vi "Periodic Tasks.vi"() -> ()   [LabVIEW 2019]
doc: "This VI runs in parallel to other tasks. It can contain as many user-defined periodic loops as you need. These can carry out PID or other sorts of timed response."
uses:
  <vilib>/Rock Robotics/Network Tables/NT Write Raw.vi
  Robot Global Data.vi
  <vilib>/vision/Image Controls.llb/IMAQ Image.ctl
  <vilib>/Rock Robotics/WPI/RobotDrive/WPI_RobotDriveArcadeDrive_Standard(NoSaturation).vi
panel:
  in  "Y axis value":dbl
  in  "X axis value":dbl
  in  "Shooting Bottom Output":dbl
  in  "Shooting Top Output":dbl
  in  "Transport Output":dbl
  in  "Intake Output":dbl
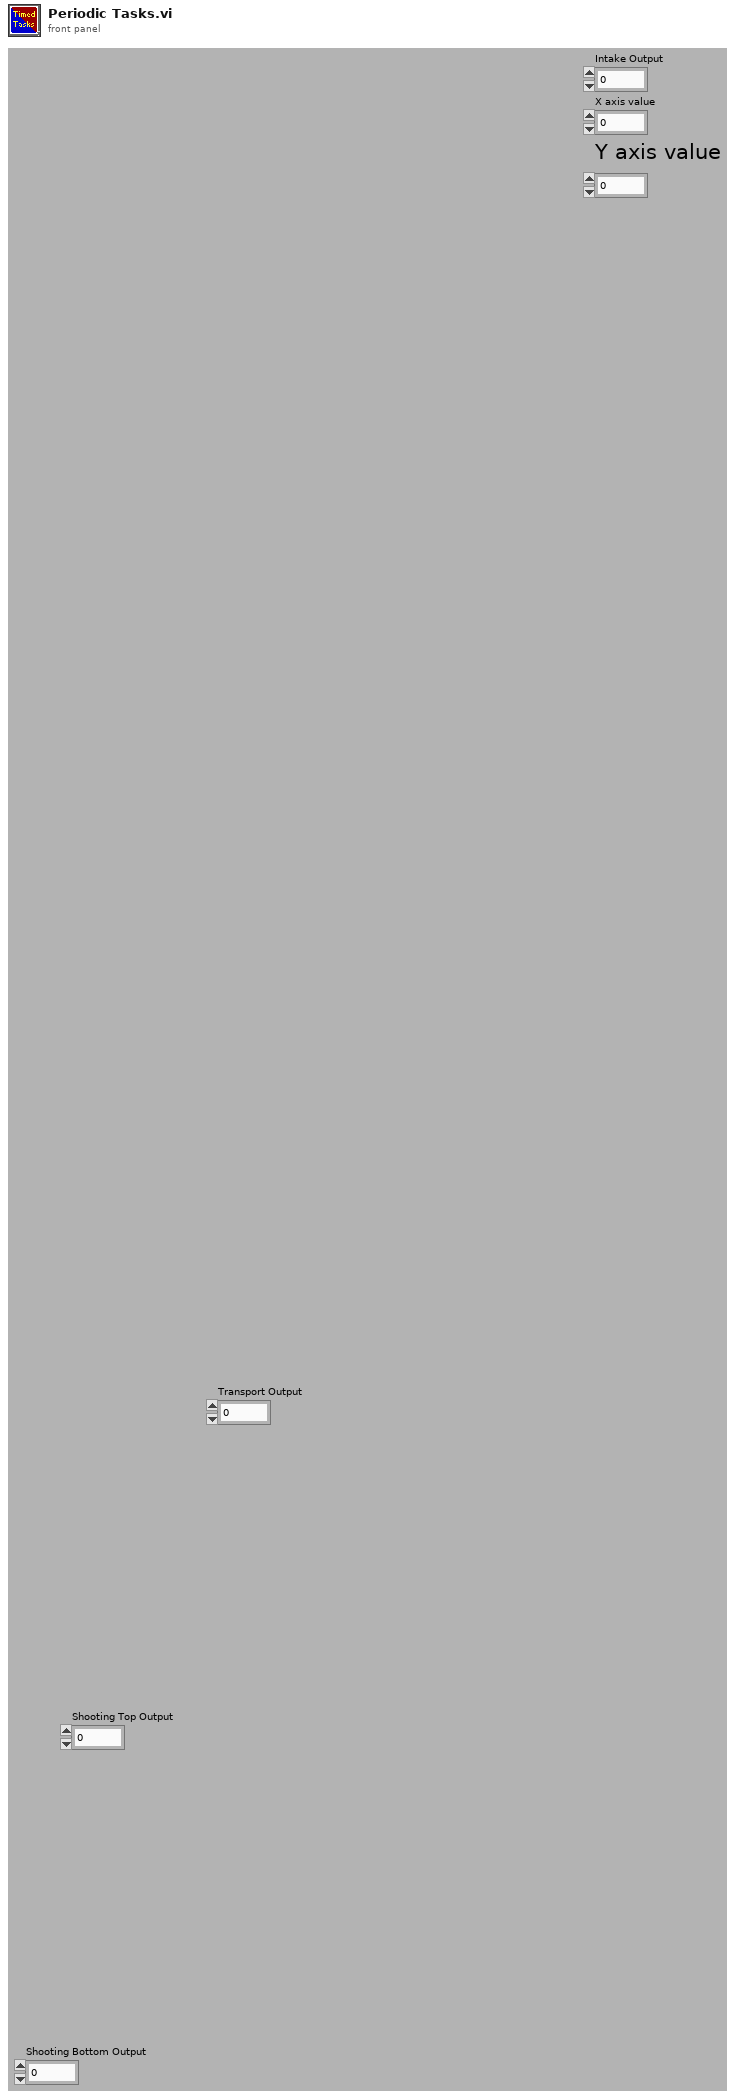
[diagram p1: front panel]
types:
  T1 = typedef "WPI_RobotDriveDevRef.ctl" = cluster{"DevStatus":errorcluster, "Motors[]":T2[], "Square Inputs":bool, "Max Output":dbl}
  T2 = typedef "WPI_MotorControlDeviceRef.ctl" = cluster{"DeviceStatus":errorcluster, "Type":T3, "PWM":cluster{"PWM Channel":T4, "DeadBand":T5}, "CAN":cluster{"Device Number":u8, "SetOutput VI Ref":variant, "GetOutput VI Ref":variant, "Enable VI Ref":variant, "Disable VI Ref":variant, "Data":variant}, "Invert":bool, "DIO PWM":cluster{"PWM \"Enable\" Channel":T4, "DIOChannel":T6, "PWM Rate":dbl}}
  T3 = typedef "WPI_MotorControlType.ctl" = enum16{"PWM", "CAN", "DIO PWM"}
  T4 = typedef "FPGA_DIOPWMChannel.ctl" = enum8{"PWM 0", "PWM 1", "PWM 2", "PWM 3", "PWM 4", "PWM 5", "PWM 6", "PWM 7", "PWM 8", "PWM 9", "PWM MXP 0", "PWM MXP 1", "PWM MXP 2", "PWM MXP 3", "PWM MXP 4", "PWM MXP 5", "PWM MXP 6", "PWM MXP 7", "PWM MXP 8", "PWM MXP 9", "Invalid"}
  T5 = typedef "WPI_PWMDeadband.ctl" = cluster{"Name":string, "maxPositivePwm":i32, "minPositivePwm":i32, "centerPwm":i32, "maxNegativePwm":i32, "minNegativePwm":i32, "angularRange":u16}
  T6 = typedef "FPGA_DIOChannel.ctl" = enum8{"DIO 0", "DIO 1", "DIO 2", "DIO 3", "DIO 4", "DIO 5", "DIO 6", "DIO 7", "DIO 8", "DIO 9", "DIO MXP 0", "DIO MXP 1", "DIO MXP 2", "DIO MXP 3", "DIO MXP 4", "DIO MXP 5", "DIO MXP 6", "DIO MXP 7", "DIO MXP 8", "DIO MXP 9", "DIO MXP 10", "DIO MXP 11", "DIO MXP 12", "DIO MXP 13", "DIO MXP 14", "DIO MXP 15", "SPI Port CS1", "SPI Port CS2", "SPI Port CS3", "SPI Port MISO", "SPI Port MOSI", "Invalid"}
  T7 = typedef "WPI_CameraDevRef.ctl" = cluster{"Camera Address":string, "CameraStatus":errorcluster}
  T8 = typedef "IMAQ Image.ctl" = refnum<image>
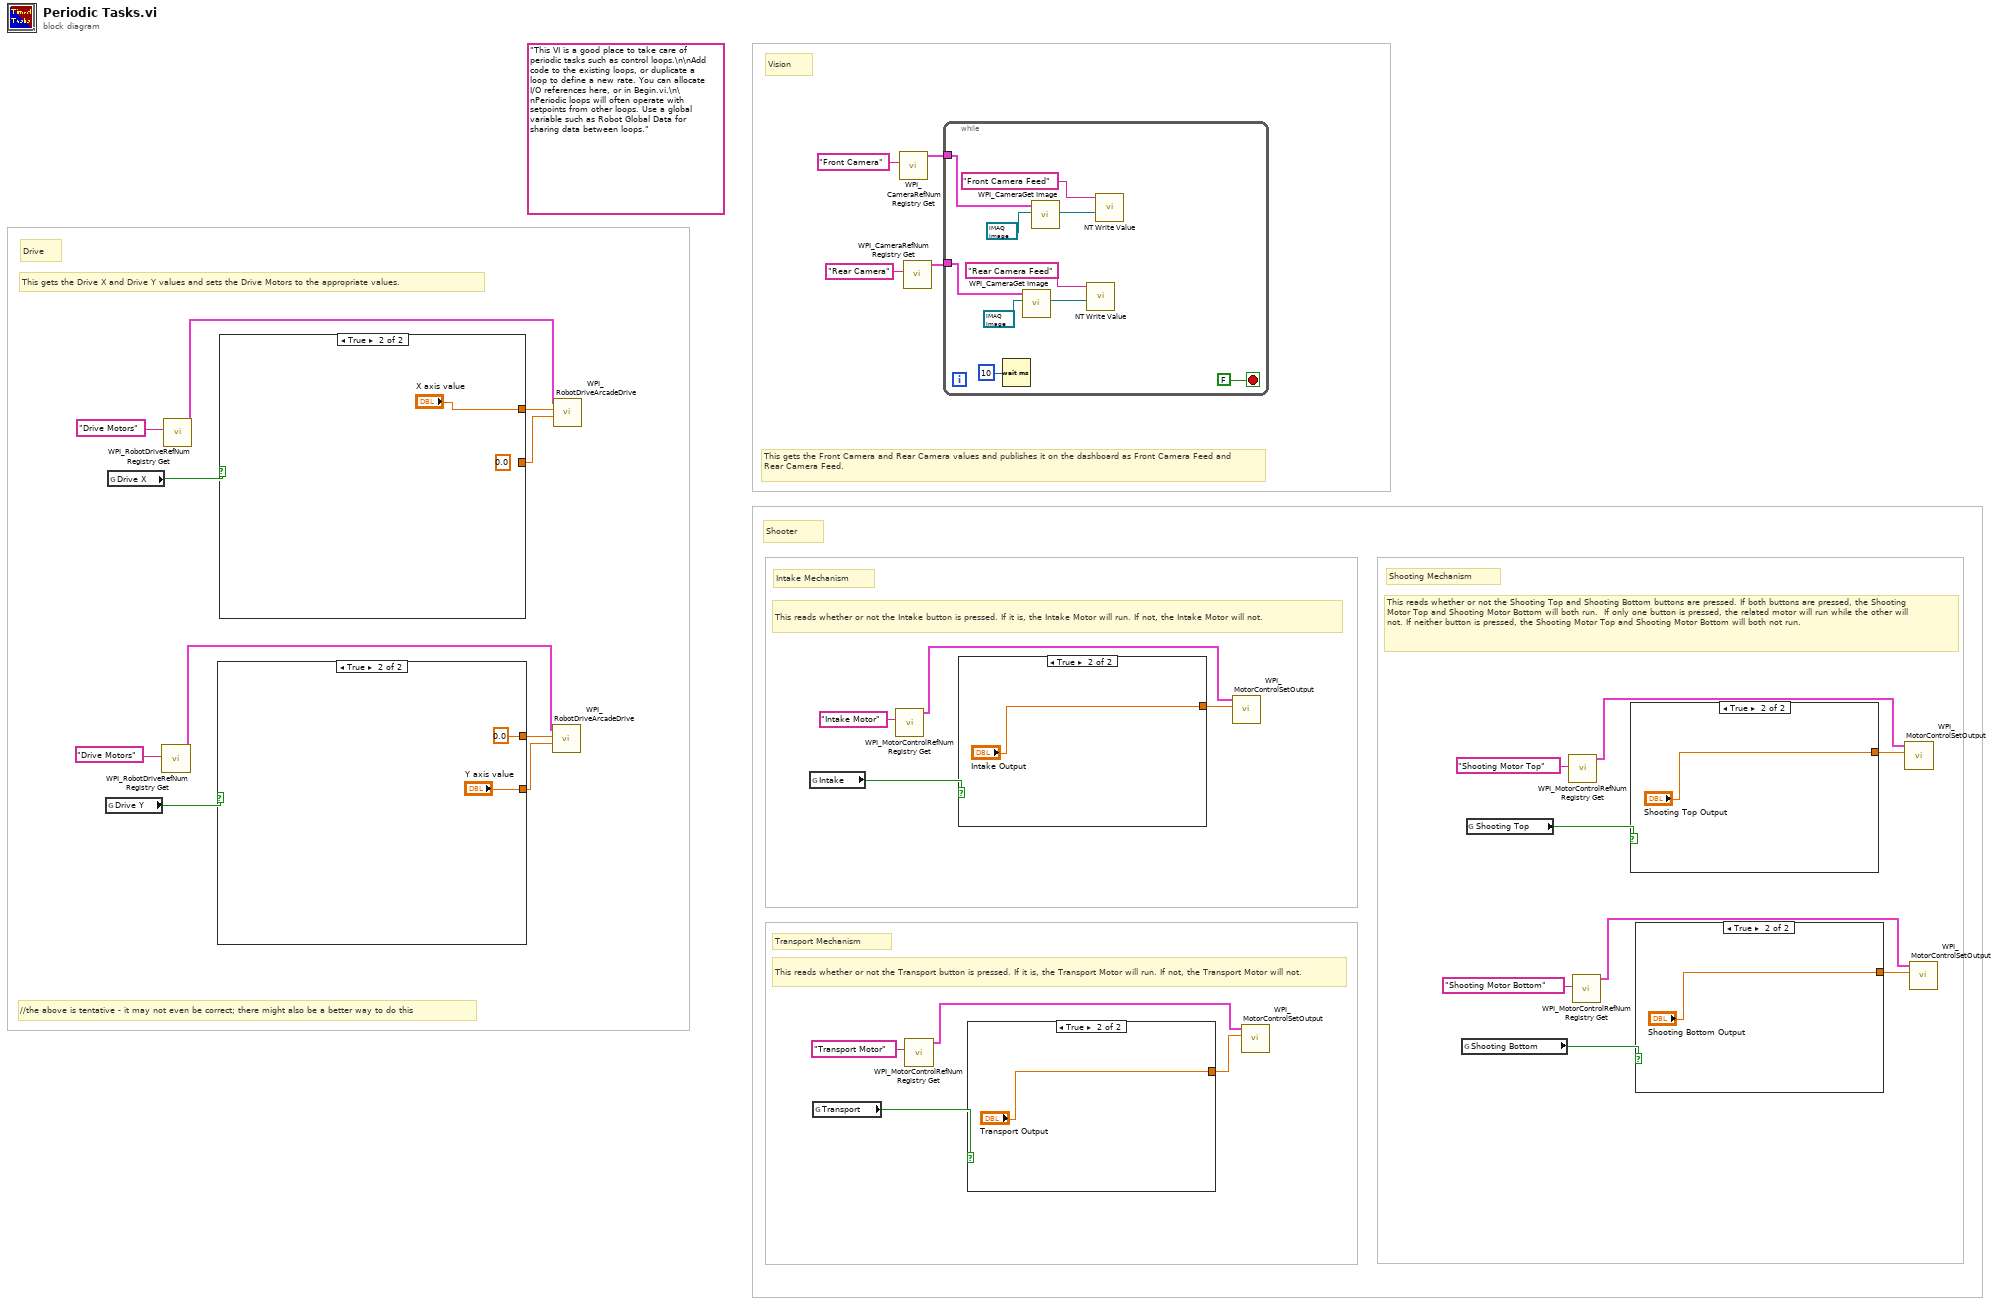
[diagram p0: block diagram]
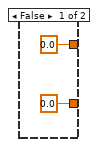
[diagram p2: hidden frame]
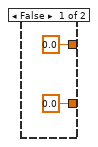
[diagram p3: hidden frame]
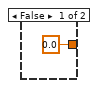
[diagram p4: hidden frame]
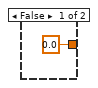
[diagram p5: hidden frame]
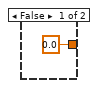
[diagram p6: hidden frame]
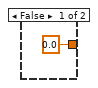
[diagram p7: hidden frame]
diagram:
  (unwired) "This VI is a good place to take care of periodic tasks such as control loops.\n\nAdd code to the existing loops, or duplicate a loop to define a new rate. You can allocate I/O references here, or in Begin.vi.\n\nPeriodic loops will often operate with setpoints from other loops. Use a global variable such as Robot Global Data for sharing data between loops."
  # "//the above is tentative - it may not even be correct; there might also be a better way to do this"
  # "This gets the Drive X and Drive Y values and sets the Drive Motors to the appropriate values."
  # "Drive"
  # "Shooter"
  # "This reads whether or not the Shooting Top and Shooting Bottom buttons are pressed. If both buttons are pressed, the Shooting Motor Top and Shooting Motor Bottom will both run.  If only one button is pressed, the related motor will run while the other will not. If neither button is pressed, the Shooting Motor Top and Shooting Motor Bottom will both not run."
  # "Shooting Mechanism"
  # "This reads whether or not the Transport button is pressed. If it is, the Transport Motor will run. If not, the Transport Motor will not."
  # "Transport Mechanism"
  # "This reads whether or not the Intake button is pressed. If it is, the Intake Motor will run. If not, the Intake Motor will not."
  # "Intake Mechanism"
  # "This gets the Front Camera and Rear Camera values and publishes it on the dashboard as Front Camera Feed and Rear Camera Feed."
  # "Vision"
  n1 = global read "Robot Global Data.vi" "Drive Y"() -> (w1:bool)
  n2 = global read "Robot Global Data.vi" "Drive X"() -> (w6:bool)
  n3 = call <vilib>:"WPI_RobotDriveRefNum Registry Get.vi"("refnum name"="Drive Motors") -> ("RobotDriveDevRef"=w4:T1)  [unwired: 9 in, 1 out]
  n4 = call <vilib>:"WPI_RobotDriveRefNum Registry Get.vi"("refnum name"="Drive Motors") -> ("RobotDriveDevRef"=w9:T1)  [unwired: 9 in, 1 out]
  n5 = case shown="True" w1 {
    tunnel: [0.0 ("X axis value") 0.0 ("X axis value")] -> w3
    tunnel: [0.0 ("Y axis value") "Y axis value"] -> w2
    frame False {
    }
    frame True {
    }
  }
  n6 = case shown="True" w6 {
    tunnel: [0.0 ("X axis value") "X axis value"] -> w8
    tunnel: [0.0 ("Y axis value") _] -> w7
    frame False {
    }
    frame True {
      (unwired) 0.0 ("Y axis value")
    }
  }
  n7 = call-poly <vilib>:"WPI_RobotDriveArcadeDrive.vi"("Y axis value"=w2, "X axis value"=w3, "RobotDriveDevRef"=w4) -> ()  [unwired: 6 in, 3 out]
  n8 = call-poly <vilib>:"WPI_RobotDriveArcadeDrive.vi"("Y axis value"=w7, "X axis value"=w8, "RobotDriveDevRef"=w9) -> ()  [unwired: 6 in, 3 out]
  n9 = global read "Robot Global Data.vi" "Intake"() -> (w26:bool)
  n10 = global read "Robot Global Data.vi" "Transport"() -> (w22:bool)
  n11 = call <vilib>:"WPI_MotorControlRefNum Registry Get.vi"("refnum name"="Intake Motor") -> ("MotorControlDevRef"=w23:T2)  [unwired: 9 in, 1 out]
  n12 = call <vilib>:"WPI_CameraRefNum Registry Get.vi"("refnum name"="Front Camera") -> ("CameraDevRef"=w29:T7)  [unwired: 9 in, 1 out]
  n13 = call <vilib>:"WPI_CameraRefNum Registry Get.vi"("refnum name"="Rear Camera") -> ("CameraDevRef"=w27:T7)  [unwired: 9 in, 1 out]
  n14 = call <vilib>:"WPI_MotorControlRefNum Registry Get.vi"("refnum name"="Transport Motor") -> ("MotorControlDevRef"=w19:T2)  [unwired: 9 in, 1 out]
  n15 = while {
    tunnel: w29 -> [w46]
    tunnel: w27 -> [w44]
    stop <- FALSE stop-if-true
    n16 = Wait (ms)(milliseconds to wait=u32 10) -> ()  [unwired: 1 out]
    n17 = call <vilib>:"WPI_CameraGet Image.vi"("Image"=T8 refnum, "CameraDevRef"=w44) -> ("Image Out"=w45:T8)  [unwired: 7 in, 2 out]
    n18 = call <vilib>:"WPI_CameraGet Image.vi"("Image"=T8 refnum, "CameraDevRef"=w46) -> ("Image Out"=w47:T8)  [unwired: 7 in, 2 out]
    n19 = call-poly <vilib>:"NT Write Value.vi"("Raw"=w45, "Name"="Rear Camera Feed") -> ()  [unwired: 9 in, 1 out]
    n20 = call-poly <vilib>:"NT Write Value.vi"("Raw"=w47, "Name"="Front Camera Feed") -> ()  [unwired: 9 in, 1 out]
  }
  n21 = case shown="True" w26 {
    tunnel: [0.0 ("Output") "Intake Output"] -> w24
    frame False {
    }
    frame True {
    }
  }
  n22 = case shown="True" w22 {
    tunnel: [0.0 ("Output") "Transport Output"] -> w20
    frame False {
    }
    frame True {
    }
  }
  n23 = call <vilib>:"WPI_MotorControlSetOutput.vi"("Output"=w24, "MotorControlDevRef"=w23) -> ()  [unwired: 7 in, 3 out]
  n24 = call <vilib>:"WPI_MotorControlSetOutput.vi"("Output"=w20, "MotorControlDevRef"=w19) -> ()  [unwired: 7 in, 3 out]
  n25 = global read "Robot Global Data.vi" "Shooting Bottom"() -> (w14:bool)
  n26 = global read "Robot Global Data.vi" "Shooting Top"() -> (w18:bool)
  n27 = call <vilib>:"WPI_MotorControlRefNum Registry Get.vi"("refnum name"="Shooting Motor Top") -> ("MotorControlDevRef"=w15:T2)  [unwired: 9 in, 1 out]
  n28 = call <vilib>:"WPI_MotorControlRefNum Registry Get.vi"("refnum name"="Shooting Motor Bottom") -> ("MotorControlDevRef"=w11:T2)  [unwired: 9 in, 1 out]
  n29 = case shown="True" w18 {
    tunnel: [0.0 ("Output") "Shooting Top Output"] -> w16
    frame False {
    }
    frame True {
    }
  }
  n30 = case shown="True" w14 {
    tunnel: [0.0 ("Output") "Shooting Bottom Output"] -> w12
    frame False {
    }
    frame True {
    }
  }
  n31 = call <vilib>:"WPI_MotorControlSetOutput.vi"("Output"=w16, "MotorControlDevRef"=w15) -> ()  [unwired: 7 in, 3 out]
  n32 = call <vilib>:"WPI_MotorControlSetOutput.vi"("Output"=w12, "MotorControlDevRef"=w11) -> ()  [unwired: 7 in, 3 out]
